vi "GetActualValues.vi"(7 "LabVIEW Web Service Request":refnum<class "Web Request.lvclass">) -> ()   [LabVIEW 2019]
uses:
  <vilib>/wsapi/Web Request.lvclass
  IndoorData_class/IndoorData.lvclass
panel:
  # "Use the Web Service Request input terminal to call the VIs on the Web Services palette. Do not remove it from the connector pane unless you don't need access to the palette."
  # "Each additional control wired to the connector pane will be available as an input in the URL. To include an indicator in terminal-mode output (the default setting), it must also be wired to the connector pane."
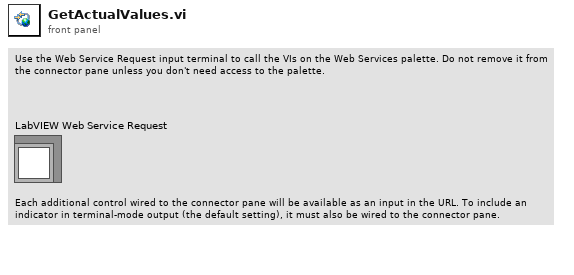
[diagram p1: front panel]
types:
  T1 = typedef "IndoorData.lvclass/ActualValues.ctl" = cluster{"Time":dbl, "Temp":dbl, "RH":dbl}
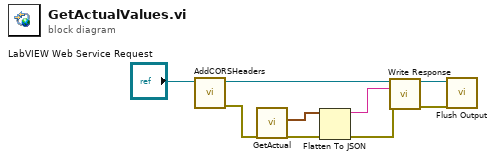
[diagram p0: block diagram]
diagram:
  n1 = call "AddCORSHeaders.vi"("LabVIEW Web Service Request"="LabVIEW Web Service Request") -> ("error out"=w6:errorcluster, "LabVIEW Web Service Request out"=w5:refnum<class "Web Request.lvclass">)  [unwired: 9 in]
  n2 = call "GetActual.vi"("error in (no error)"=w6) -> ("Actual"=w3:T1, "error out"=w4:errorcluster)  [unwired: 17 in]
  n3 = Flatten To JSON(anything=w3, error in (no error)=w4) -> (JSON string=w2:string, 11:w1:errorcluster)  [unwired: 1 in]
  n4 = call <vilib>:"Write Response.vi"("LabVIEW Web Service Request"=w5, "response string"=w2, "error in (no error)"=w1) -> ("LabVIEW Web Service Request out"=w9:refnum<class "Web Request.lvclass">, "error out"=w8:errorcluster)  [unwired: 11 in]
  n5 = call <vilib>:"Flush Output.vi"("LabVIEW Web Service Request"=w9, "error in (no error)"=w8) -> ()  [unwired: 12 in, 2 out]
